vi "AverageSignal.vi"(11 "Data in Volts":dbl[][][](array[numeric])) -> (3 "Array":dbl[][](array[numeric]))   [LabVIEW 2018]
panel:
  out "element":i32
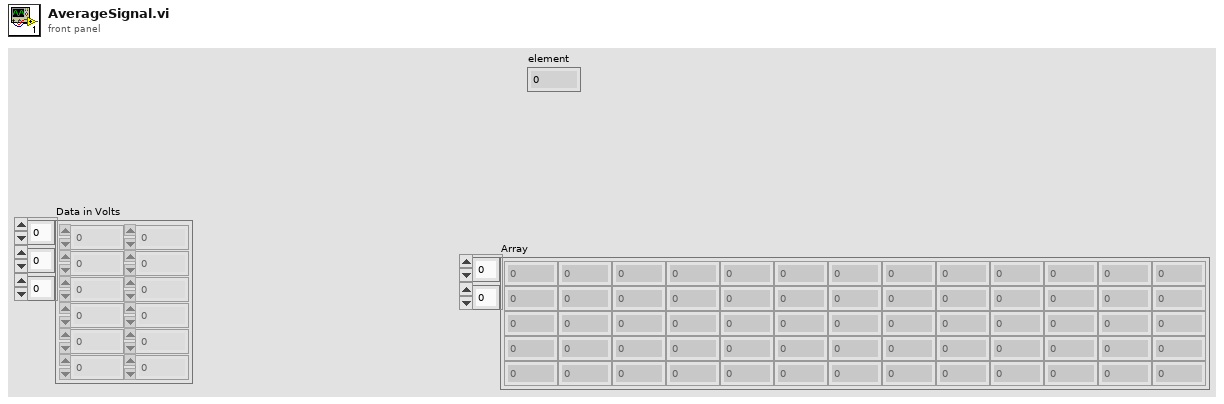
[diagram p1: front panel]
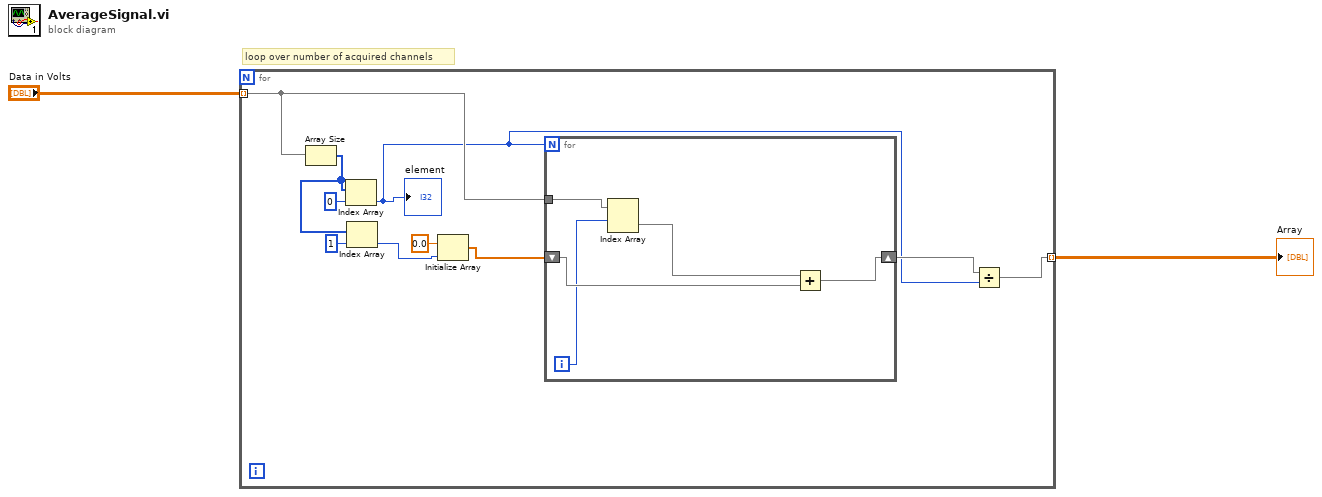
[diagram p0: block diagram]
diagram:
  # "loop over number of acquired channels"
  n1 = for {
    tunnel: "Data in Volts" -> [w11] mode=indexing
    tunnel: [w4] -> w1 mode=indexing
    n2 = Array Size(array=w11) -> (size(s)=w8:i32[])
    n3 = Index Array(array=w8, index=0) -> (element=w3:i32)
    "element" <- w3
    n4 = Index Array(array=w8, index=1) -> (element=w6:i32)
    n5 = Initialize Array(0.0 ("element"), w6) -> (w9:dbl[])
    n6 = for {
      N: w3 -> [_]
      tunnel: w11 -> [w17]
      shift-right: [w16] -> w5
      shift-left: w9 -> [w15]
      i -> [w13]
      n7 = Index Array(array=w17, index (row)=w13) -> (element=w14:dbl[])  [unwired: 1 in]
      n8 = Add(x=w14, y=w15) -> (x+y=w16:dbl[])
    }
    n9 = Divide(x=w5, y=w3) -> (x/y=w4:dbl[])
  }
  "Array" <- w1
